vi "VIP_Post-Install Custom Action.vi"(10 "Variant":variant) -> (0 "error out":errorcluster)   [LabVIEW 2021]
uses:
  <vilib>/regexp/Match Regular Expression.xnode
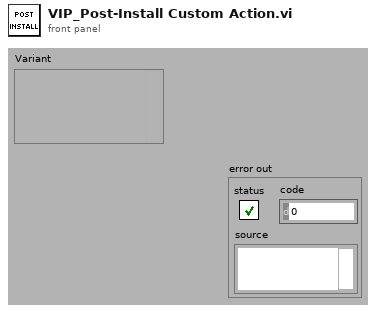
[diagram p1: front panel]
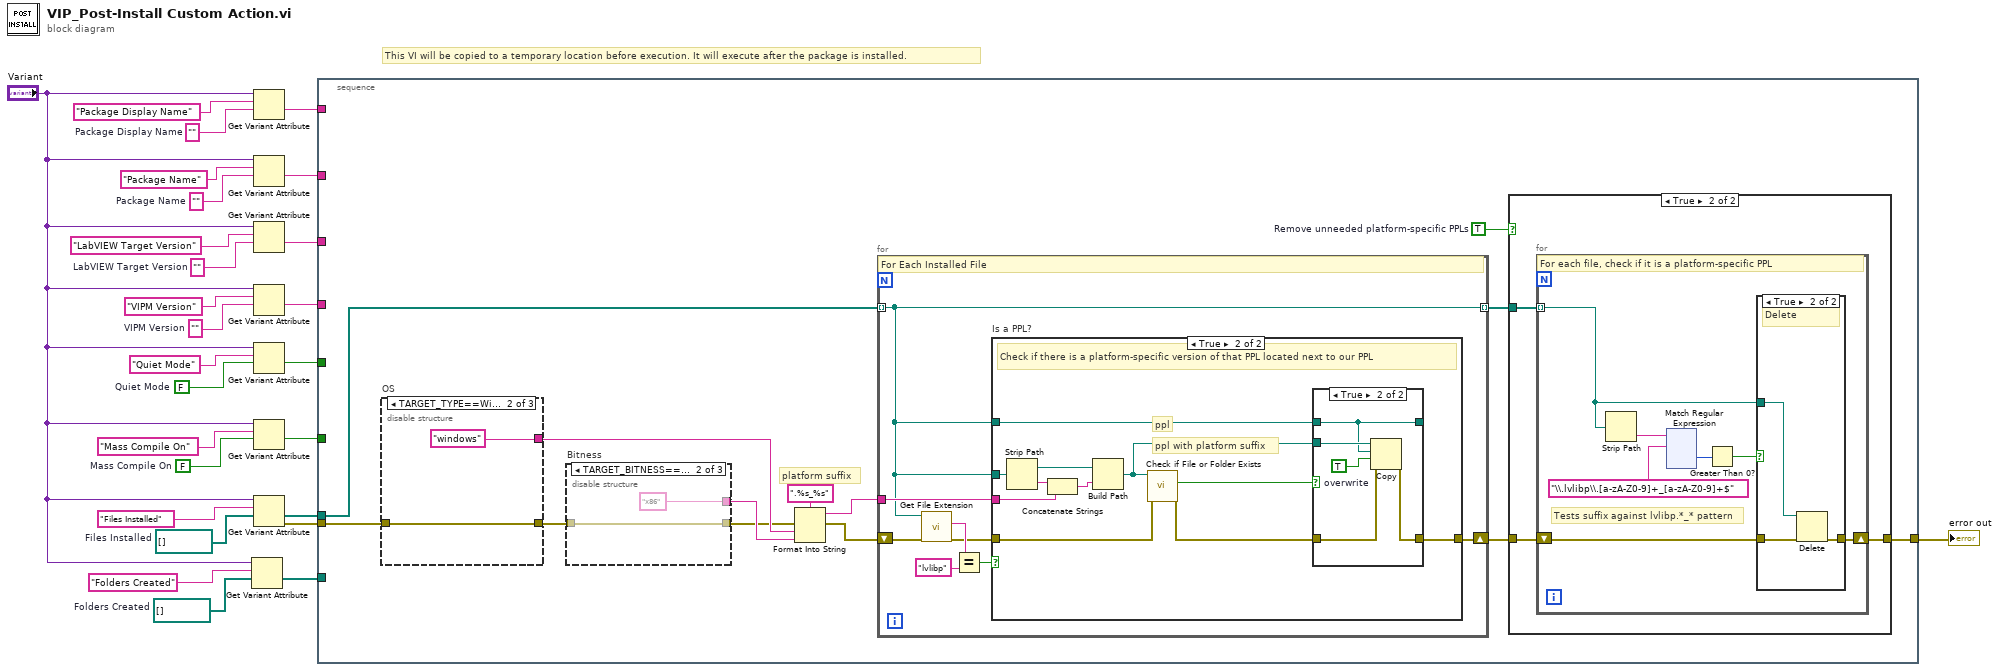
[diagram p0: block diagram]
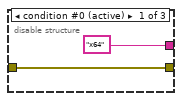
[diagram p2: hidden frame]
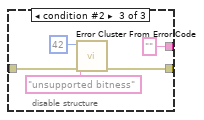
[diagram p3: hidden frame]
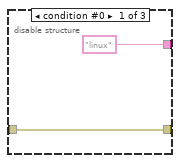
[diagram p4: hidden frame]
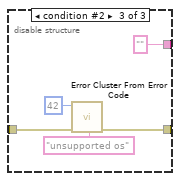
[diagram p5: hidden frame]
diagram:
  w3 = path[] []  # Folders Created
  w4 = path[] []  # Files Installed
  w10 = FALSE  # Mass Compile On
  w11 = ""  # Package Display Name
  w18 = FALSE  # Quiet Mode
  w21 = ""  # VIPM Version
  w23 = ""  # LabVIEW Target Version
  w25 = ""  # Package Name
  # "This VI will be copied to a temporary location before execution. It will execute after the package is installed."
  n1 = Get Variant Attribute(Variant="Variant", name="Folders Created", default value (empty Variant)=w3) -> (value=w8:path[])  [unwired: 1 in, 3 out]
  n2 = Get Variant Attribute(Variant="Variant", name="Package Display Name", default value (empty Variant)=w11) -> (value=w17:string)  [unwired: 1 in, 3 out]
  n3 = Get Variant Attribute(Variant="Variant", name="Package Name", default value (empty Variant)=w25) -> (value=w16:string)  [unwired: 1 in, 3 out]
  n4 = Get Variant Attribute(Variant="Variant", name="LabVIEW Target Version", default value (empty Variant)=w23) -> (value=w15:string)  [unwired: 1 in, 3 out]
  n5 = Get Variant Attribute(Variant="Variant", name="VIPM Version", default value (empty Variant)=w21) -> (value=w14:string)  [unwired: 1 in, 3 out]
  n6 = Get Variant Attribute(Variant="Variant", name="Quiet Mode", default value (empty Variant)=w18) -> (value=w13:bool)  [unwired: 1 in, 3 out]
  n7 = Get Variant Attribute(Variant="Variant", name="Mass Compile On", default value (empty Variant)=w10) -> (value=w12:bool)  [unwired: 1 in, 3 out]
  n8 = Get Variant Attribute(Variant="Variant", name="Files Installed", default value (empty Variant)=w4) -> (value=w7:path[], error out=w2:errorcluster)  [unwired: 1 in, 2 out]
  n9 = stacked-sequence {
    tunnel: w17 -> [_]
    tunnel: w16 -> [_]
    tunnel: w15 -> [_]
    tunnel: w14 -> [_]
    tunnel: w13 -> [_]
    tunnel: w12 -> [_]
    tunnel: w7 -> [w40]
    tunnel: w8 -> [_]
    tunnel: w2 -> [w38]
    tunnel: [w29] -> w1
    frame #0 {
      w31 = TRUE  # Remove unneeded platform-specific PPLs
      # "platform suffix"
      n10 = disable-structure "OS" shown="TARGET_TYPE==Windows" {
        disable-tunnel: ["linux" "windows" ""] -> w37
        disable-tunnel: [w50 w52 w55] -> w39
        disable-tunnel: w38 -> [w50 w52 w54]
        frame condition #0 {
        }
        frame condition #1 (active) {
        }
        frame condition #2 {
          n11 = call <vilib>:"Error Cluster From Error Code.vi"("error in (no error)"=w54, "error message (\"\")"="unsupported os" ("error message (\"\")"), "error code (0)"=42) -> ("error out"=w55:errorcluster)  [unwired: 6 in]
        }
      }
      n12 = disable-structure "Bitness" shown="TARGET_BITNESS==32" {
        disable-tunnel: ["x64" "x86" ""] -> w36
        disable-tunnel: w39 -> [w41 w43 w46]
        disable-tunnel: [w41 w43 w45] -> w33
        frame condition #0 (active) {
        }
        frame condition #1 {
        }
        frame condition #2 {
          n13 = call <vilib>:"Error Cluster From Error Code.vi"("error in (no error)"=w46, "error message (\"\")"="unsupported bitness" ("error message (\"\")"), "error code (0)"=42) -> ("error out"=w45:errorcluster)  [unwired: 6 in]
        }
      }
      n14 = Format Into String(format string=".%s_%s", error in=w33, w37, w36) -> (resulting string=w34:string, error out=w32:errorcluster)  [unwired: 1 in]
      n15 = for {
        tunnel: w40 -> [w59] mode=indexing
        tunnel: w34 -> [w64]
        shift-right: [w60] -> w30
        shift-left: w32 -> [w61]
        tunnel: [w59] -> w28 mode=indexing
        # "For Each Installed File"
        n16 = call <vilib>:"Get File Extension.vi"("error in (no error)"=w61, "file"=w59) -> ("error out"=w62:errorcluster, "lowercase file extension"=w66:string)  [unwired: 5 in, 3 out]
        n17 = Equal?(x=w66, y="lvlibp" ("lowercase file extension")) -> (x = y?=w63:bool)
        n18 = case "Is a PPL?" shown="True" w63 {
          tunnel: w59 -> [_ w78]
          tunnel: w64 -> [_ w76]
          tunnel: w62 -> [w67 w69]
          tunnel: [w67 w68] -> w60
          tunnel: w59 -> [_ w73]
          frame False {
          }
          frame True {
            # "ppl"
            # "ppl with platform suffix"
            # "Check if there is a platform-specific version of that PPL located next to our PPL"
            n19 = Strip Path(path=w78) -> (stripped path=w75:path, name=w77:string)
            n20 = Concatenate Strings(w77, w76) -> (w74:string)
            n21 = Build Path(base path=w75, name or relative path=w74) -> (appended path=w72:path)
            n22 = call <vilib>:"Check if File or Folder Exists.vi"("error in (no error)"=w69, "path"=w72) -> ("error out"=w70:errorcluster, "file or folder exists?"=w71:bool)  [unwired: 7 in, 1 out]
            n23 = case shown="True" w71 {
              tunnel: [w80 w84] -> w68
              tunnel: w70 -> [w80 w83]
              tunnel: w73 -> [w79 w81]
              tunnel: w72 -> [_ w85]
              tunnel: [w79 w81] -> _
              frame False {
              }
              frame True {
                w82 = TRUE  # overwrite
                n24 = Copy(8:w83, 9:w82, 10:w81, 11:w85) -> (0:w84:errorcluster)  [unwired: 1 in, 2 out]
              }
            }
          }
        }
      }
      n25 = case shown="True" w31 {
        tunnel: w30 -> [w86 w88]
        tunnel: [w86 w87] -> w29
        tunnel: w28 -> [_ w89]
        frame False {
        }
        frame True {
          n26 = for {
            tunnel: w89 -> [w90] mode=indexing
            shift-right: [w91] -> w87
            shift-left: w88 -> [w92]
            # "Tests suffix against lvlibp.*_* pattern"
            # "For each file, check if it is a platform-specific PPL"
            n27 = Strip Path(path=w90) -> (name=w95:string)  [unwired: 1 out]
            n28 = xnode "Match Regular Expression"("input string"=w95, "regular expression"="\\.lvlibp\\.[a-zA-Z0-9]+_[a-zA-Z0-9]+$") -> ("offset past match"=w94:i32)  [unwired: 4 in, 4 out]
            n29 = Greater Than 0?(x=w94) -> (x > 0?=w93:bool)
            n30 = case shown="True" w93 {
              tunnel: w92 -> [w97 w100]
              tunnel: [w97 w99] -> w91
              tunnel: w90 -> [_ w98]
              frame False {
              }
              frame True {
                # "Delete"
                n31 = Delete(path (use dialog)=w98, error in=w100) -> (error out=w99:errorcluster)  [unwired: 3 in, 2 out]
              }
            }
          }
        }
      }
    }
  }
  "error out" <- w1
